vi "Action.vi"(8 "error in (no error)":errorcluster, 10 "OOQMH in":refnum<class "OOQMH.lvclass">, 11 "Message in":refnum<class "Message.lvclass">) -> (0 "error out":errorcluster, 2 "OOQMH out":refnum<class "OOQMH.lvclass">, 3 "Message out":refnum<class "Message.lvclass">)   [LabVIEW 2024, in "OOQMH.lvlib" / "Message.lvclass"]
uses:
  Message.lvclass
  OOQMH/OOQMH.lvclass
  Message.lvclass/Message.ctl
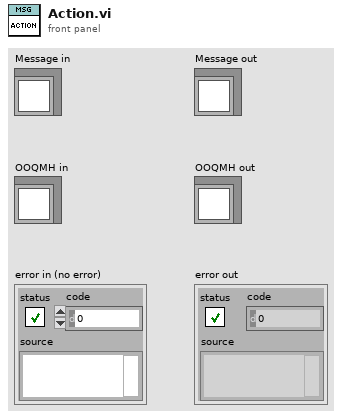
[diagram p1: front panel]
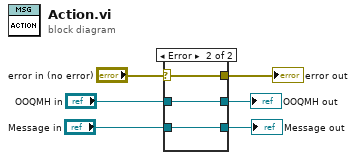
[diagram p0: block diagram]
diagram:
  n1 = case shown="Error" "error in (no error)" {
    selector: "error in (no error)" -> [w8 w12]
    tunnel: [w8 w12] -> w5
    tunnel: [w9 w11] -> w3
    tunnel: "Message in" -> [w9 w11]
    tunnel: [w7 w10] -> w2
    tunnel: "OOQMH in" -> [w7 w10]
    frame No Error {
    }
    frame Error {
    }
  }
  "error out" <- w5
  "Message out" <- w3
  "OOQMH out" <- w2
